vi "gateway打开历史文件.vi"() -> ()   [LabVIEW 2012]
panel:
  out "亮度":sgl[](graph)
  out "温度":sgl[][](graph)
  in  "路径":path
  in  "停止":bool
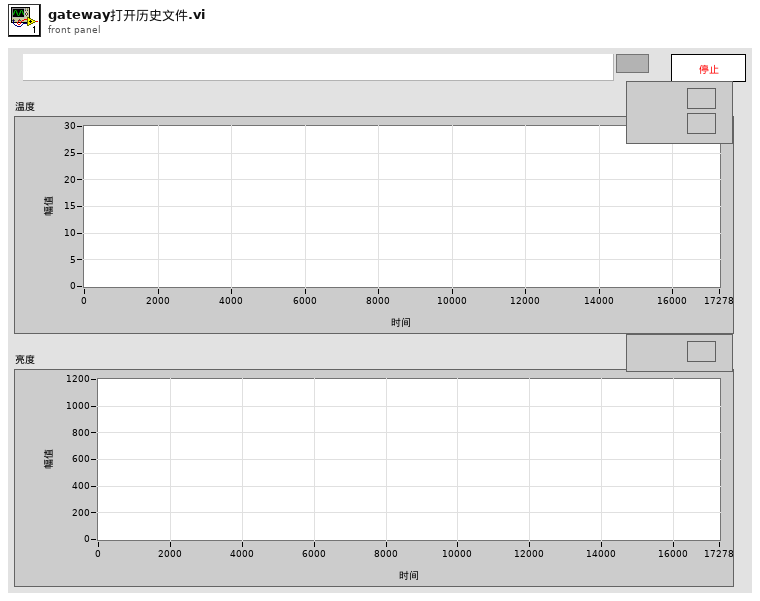
[diagram p1: front panel]
types:
  T1 = enum16{"open", "open or create", "create or replace", "create", "open (read-only)"}
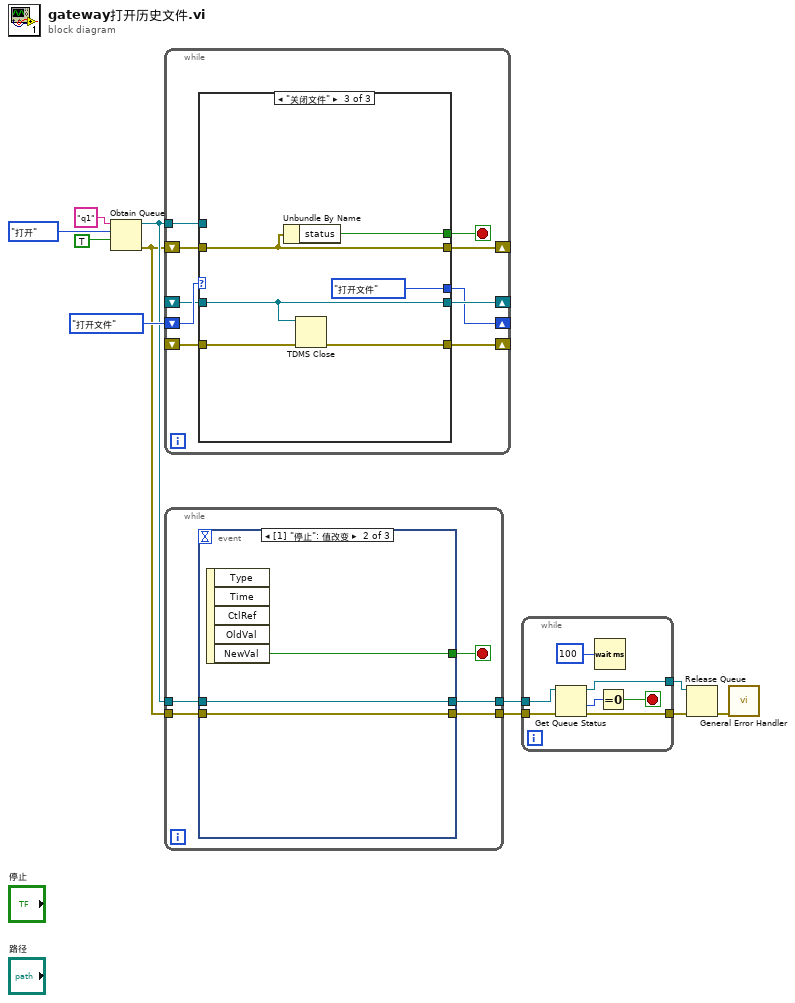
[diagram p0: block diagram]
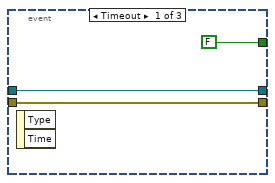
[diagram p2: hidden frame]
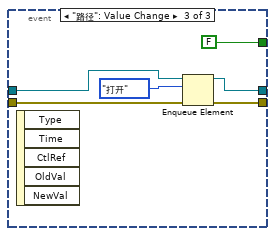
[diagram p3: hidden frame]
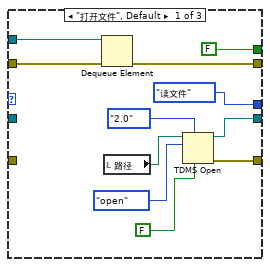
[diagram p4: hidden frame]
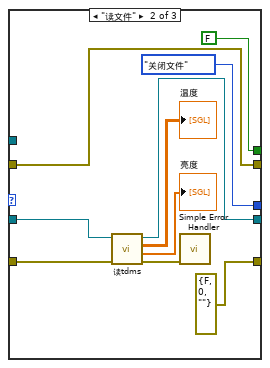
[diagram p5: hidden frame]
diagram:
  n1 = Obtain Queue(name (unnamed)="q1" ("名称（未命名）"), element data type=enum16{"打开"}."打开", create if not found? (T)=TRUE ("如未找到是否创建？(T)")) -> (queue out=w7:refnum<queue>, error out=w1:errorcluster)  [unwired: 2 in, 1 out]
  n2 = while {
    shift-right: [w21] -> _
    shift-left: _ -> [w17]
    shift-right: [w20] -> _
    shift-left: _ -> [w16]
    shift-right: [w18] -> _
    shift-left: enum16{"打开文件", "读文件", "关闭文件"}."打开文件" -> [w19]
    tunnel: w7 -> [w15]
    shift-right: [w14] -> _
    shift-left: w1 -> [w12]
    stop <- w13 stop-if-true
    n3 = case shown="\"关闭文件\"" w19 {
      tunnel: [w29 w39 w46] -> w21
      tunnel: [w28 errorcluster {"status"=FALSE, "code"=0, "source"=""} ("error out") w45] -> w20
      tunnel: [enum16{"打开文件", "读文件", "关闭文件"}."读文件" enum16{"打开文件", "读文件", "关闭文件"}."关闭文件" enum16{"打开文件", "读文件", "关闭文件"}."打开文件"] -> w18
      tunnel: w17 -> [_ w41 w46]
      tunnel: w16 -> [_ w40 w48]
      tunnel: w15 -> [w24 _ _]
      tunnel: [w22 w36 w43] -> w14
      tunnel: [FALSE ("status") FALSE ("status") w44] -> w13
      tunnel: w12 -> [w23 w36 w43]
      frame "打开文件", Default {
        n4 = Dequeue Element(queue=w24, error in (no error)=w23) -> (error out=w22:errorcluster)  [unwired: 1 in, 3 out]
        n5 = local read "路径"() -> (w25:path)
        n6 = TDMS Open(6:FALSE ("禁用缓冲？(T)"), 7:enum16{"1.0", "2.0"}."2.0" ("文件格式版本(2.0)"), 10:T1."open" ("操作(0:open)"), 11:w25) -> (0:w28:errorcluster, 3:w29:refnum<k34>)  [unwired: 2 in]
      }
      frame "读文件" {
        n7 = call "读tdms.vi"("错误输入（无错误）"=w40, "引用句柄输入"=w41) -> ("错误输出"=w34:errorcluster, "数据"=→"亮度":sgl[], "添加的数组"=→"温度":sgl[][], "引用句柄输出"=w39:refnum<k34>)  [unwired: 6 in]
        n8 = call <vilib>:"Simple Error Handler.vi"("error in (no error)"=w34) -> ()  [unwired: 4 in, 5 out]
      }
      frame "关闭文件" {
        n9 = Unbundle By Name(w43) -> ("status"=w44:bool)
        n10 = TDMS Close(8:w48, 11:w46) -> (0:w45:errorcluster)  [unwired: 1 out]
      }
    }
  }
  n11 = while {
    tunnel: w7 -> [w53]
    tunnel: w1 -> [w52]
    tunnel: [w51] -> w5
    tunnel: [w50] -> w6
    stop <- w49 stop-if-true
    n12 = event shown="[1] \"停止\": 值改变" {
      selector: _ -> [_ _ _]
      dyn-events: _ -> [_ _ _]
      timeout: _ -> [_ _ _]
      tunnel: [FALSE ("NewVal") w59 FALSE ("NewVal")] -> w49
      tunnel: w53 -> [w56 w58 w65]
      tunnel: w52 -> [w55 w57 w62]
      tunnel: [w55 w57 w61] -> w51
      tunnel: [w56 w58 w64] -> w50
      event Timeout {
        n13 = event-data() -> ()  [unwired: 1 in, 2 out]
      }
      event "停止": Value Change {
        n14 = event-data() -> ("NewVal"=w59:bool)  [unwired: 1 in, 4 out]
      }
      event "路径": Value Change {
        n15 = event-data() -> ()  [unwired: 1 in, 5 out]
        n16 = Enqueue Element(queue=w65, element=enum16{"打开"}."打开" ("元素"), error in (no error)=w62) -> (queue out=w64:refnum<queue>, error out=w61:errorcluster)  [unwired: 1 in, 1 out]
      }
    }
  }
  n17 = while {
    tunnel: w6 -> [w71]
    tunnel: w5 -> [w70]
    tunnel: [w69] -> w4
    tunnel: [w68] -> w3
    stop <- w67 stop-if-true
    n18 = Get Queue Status(queue=w71, error in (no error)=w70) -> (queue out=w69:refnum<queue>, # pending insert=w66:i32, error out=w68:errorcluster)  [unwired: 1 in, 5 out]
    n19 = Wait (ms)(milliseconds to wait=u32 100 ("等待时间（毫秒）")) -> ()  [unwired: 1 out]
    n20 = Equal To 0?(x=w66) -> (x = 0?=w67:bool)
  }
  n21 = Release Queue(queue=w4, error in (no error)=w3) -> (error out=w2:errorcluster)  [unwired: 1 in, 2 out]
  n22 = call <vilib>:"General Error Handler.vi"("error in (no error)"=w2) -> ()  [unwired: 10 in, 5 out]
